vi "Read Calculation Results.vi"(0 "VISA resource name":refnum<visa-resource-name>, 5 "Calculate Option (0: Read Math Calculation)":i32(ring) items=["Read Math Calculation", "Recalculate Math Calculation", "Read Buffer Data Calculation", "Read Limit Tests"], 11 "error in (no error)":errorcluster) -> (3 "Limit1 Test Failed":bool, 4 "VISA resource name out":refnum<visa-resource-name>, 6 "Math Calculation Result":string="0", 8 "Buffer Data Calculation Result":dbl format="%.6e", 10 "Composite Result":bool, 14 "Limit2 Test Failed":bool, 15 "error out":errorcluster)   [LabVIEW 2016, in "Keithley 6517.lvlib"]
doc: "Performs CALC 1, CALC2 or CALC3 calculate operation and reads the result.\n\n<B>Note:</B>\n(1) Composite Limit Result is not compatible with <B>model 6514</B>. When reading limit tests, Composite Limit Result will always reaad -1 indicating invalid or no data.\n(2) You must first enable selected calculation (CALC1, CALC2, or CALC3) and run <B>Initiate</B> VI in Low-level Data."
uses:
  <instrlib>/Keithley 6517/Keithley 6517.lvlib
panel:
  # "Limit Tests Results"
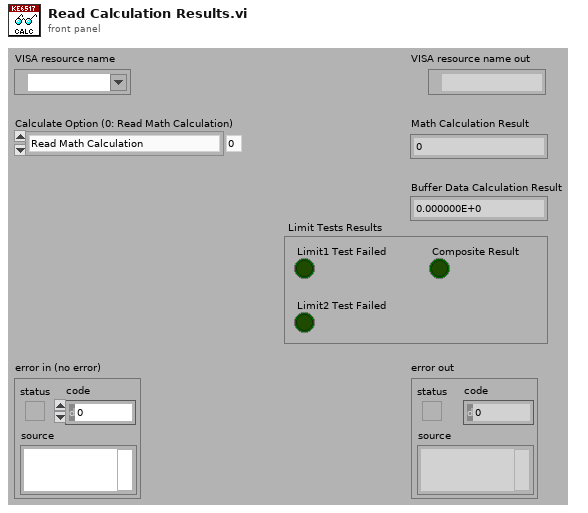
[diagram p1: front panel]
types:
  T1 = typedef "Keithley 6517.lvlib/Extended User Data.ctl" = cluster{"Instrument Model":i32}
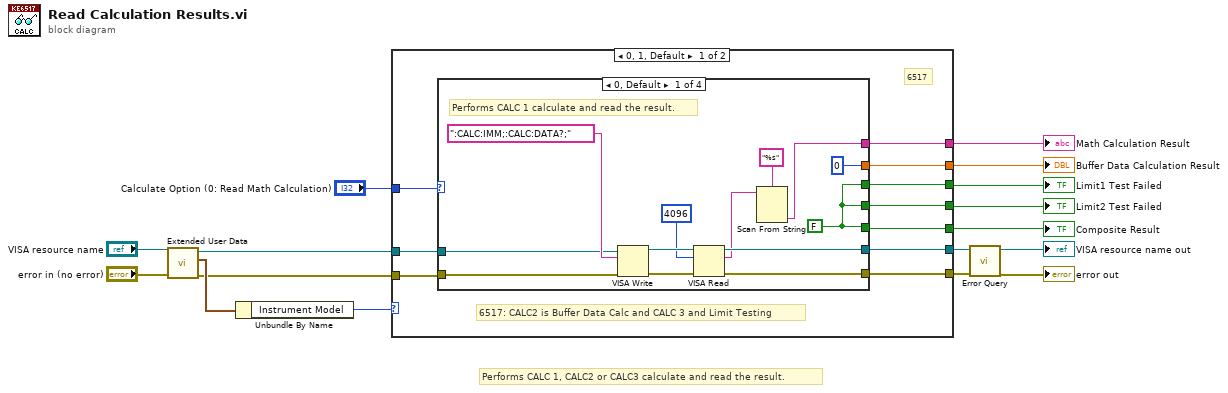
[diagram p0: block diagram]
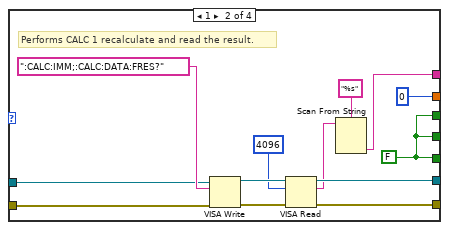
[diagram p2: hidden frame]
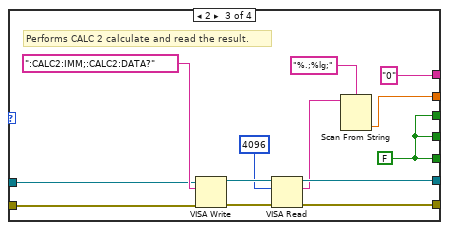
[diagram p3: hidden frame]
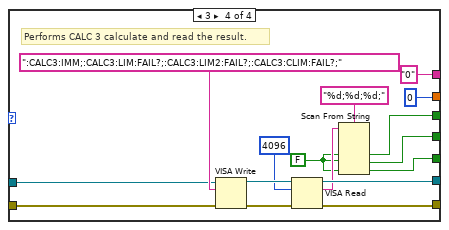
[diagram p4: hidden frame]
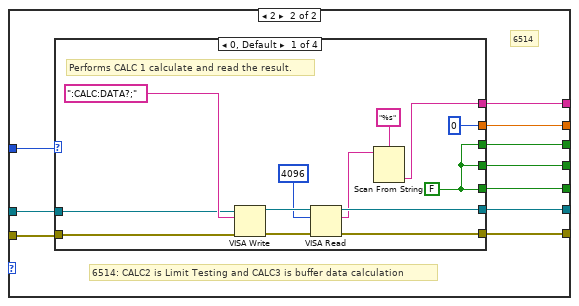
[diagram p5: hidden frame]
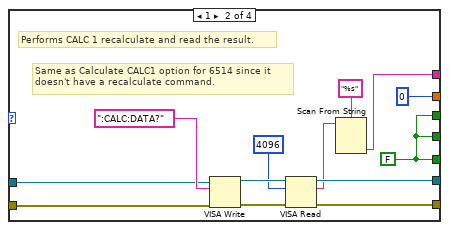
[diagram p6: hidden frame]
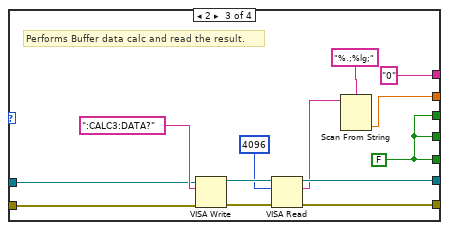
[diagram p7: hidden frame]
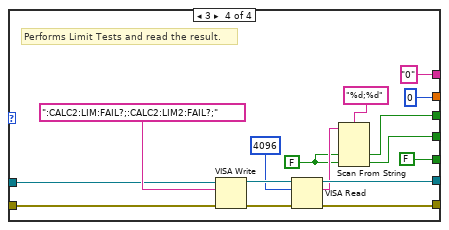
[diagram p8: hidden frame]
diagram:
  # "Performs CALC 1, CALC2 or CALC3 calculate and read the result."
  n1 = call <instrlib>:"Extended User Data.vi"("error in (no error)"="error in (no error)", "VISA resource name"="VISA resource name") -> ("error out"=w9:errorcluster, "User Data Out"=w10:T1, "VISA resource name out"=w8:refnum<visa-resource-name>)  [unwired: 7 in]
  n2 = Unbundle By Name(w10) -> ("Instrument Model"=w7:i32)
  n3 = case shown="0, 1, Default" w7 {
    tunnel: "Calculate Option (0: Read Math Calculation)" -> [w26 w91]
    tunnel: [w25 w90] -> w13
    tunnel: [w24 w89] -> w12
    tunnel: [w23 w88] -> w11
    tunnel: [w22 w87] -> w4
    tunnel: w9 -> [w21 w86]
    tunnel: w8 -> [w20 w85]
    tunnel: [w19 w84] -> w3
    tunnel: [w18 w83] -> w2
    tunnel: [w17 w82] -> w1
    frame 0, 1, Default {
      # "6517"
      # "6517: CALC2 is Buffer Data Calc and CALC 3 and Limit Testing"
      n4 = case shown="0, Default" w26 {
        tunnel: w21 -> [w34 w47 w60 w76]
        tunnel: [w33 w46 w59 w75] -> w25
        tunnel: [w32 w45 w58 w74] -> w24
        tunnel: [w31 w44 "0" "0"] -> w23
        tunnel: [0 0 w55 0] -> w22
        tunnel: w20 -> [w28 w41 w54 w70]
        tunnel: [w27 w40 w53 w68] -> w19
        tunnel: [w27 w40 w53 w67] -> w18
        tunnel: [w27 w40 w53 w66] -> w17
        frame 0, Default {
          w27 = FALSE
          # "Performs CALC 1 calculate and read the result."
          n5 = VISA Write(VISA resource name=w28, write buffer=":CALC:IMM;:CALC:DATA?;", error in (no error)=w34) -> (VISA resource name out=w38:refnum<visa-resource-name>, error out=w39:errorcluster)  [unwired: 1 out]
          n6 = VISA Read(VISA resource name=w38, byte count=u32 4096, error in (no error)=w39) -> (VISA resource name out=w33:refnum<visa-resource-name>, read buffer=w29:string, error out=w32:errorcluster)  [unwired: 1 out]
          n7 = Scan From String(format string="%s", input string=w29) -> (output 1=w31:string)  [unwired: 3 in, 3 out]
        }
        frame 1 {
          w40 = FALSE
          # "Performs CALC 1 recalculate and read the result."
          n8 = VISA Write(VISA resource name=w41, write buffer=":CALC:IMM;:CALC:DATA:FRES?", error in (no error)=w47) -> (VISA resource name out=w51:refnum<visa-resource-name>, error out=w52:errorcluster)  [unwired: 1 out]
          n9 = VISA Read(VISA resource name=w51, byte count=u32 4096, error in (no error)=w52) -> (VISA resource name out=w46:refnum<visa-resource-name>, read buffer=w42:string, error out=w45:errorcluster)  [unwired: 1 out]
          n10 = Scan From String(format string="%s", input string=w42) -> (output 1=w44:string)  [unwired: 3 in, 3 out]
        }
        frame 2 {
          w53 = FALSE
          # "Performs CALC 2 calculate and read the result."
          n11 = VISA Write(VISA resource name=w54, write buffer=":CALC2:IMM;:CALC2:DATA?", error in (no error)=w60) -> (VISA resource name out=w64:refnum<visa-resource-name>, error out=w65:errorcluster)  [unwired: 1 out]
          n12 = VISA Read(VISA resource name=w64, byte count=u32 4096, error in (no error)=w65) -> (VISA resource name out=w59:refnum<visa-resource-name>, read buffer=w57:string, error out=w58:errorcluster)  [unwired: 1 out]
          n13 = Scan From String(format string="%.;%lg;", input string=w57) -> (output 1=w55:dbl)  [unwired: 3 in, 3 out]
        }
        frame 3 {
          w69 = FALSE
          # "Performs CALC 3 calculate and read the result."
          n14 = VISA Write(VISA resource name=w70, write buffer=":CALC3:IMM;:CALC3:LIM:FAIL?;:CALC3:LIM2:FAIL?;:CALC3:CLIM:FAIL?;", error in (no error)=w76) -> (VISA resource name out=w80:refnum<visa-resource-name>, error out=w81:errorcluster)  [unwired: 1 out]
          n15 = VISA Read(VISA resource name=w80, byte count=u32 4096, error in (no error)=w81) -> (VISA resource name out=w75:refnum<visa-resource-name>, read buffer=w71:string, error out=w74:errorcluster)  [unwired: 1 out]
          n16 = Scan From String(format string="%d;%d;%d;", input string=w71, default 1=w69, default 2=w69, default 3=w69) -> (output 1=w68:bool, output 2=w67:bool, output 3=w66:bool)  [unwired: 2 in, 3 out]
        }
      }
    }
    frame 2 {
      # "6514"
      # "6514: CALC2 is Limit Testing and CALC3 is buffer data calculation"
      n17 = case shown="0, Default" w91 {
        tunnel: w86 -> [w94 w106 w125 w141]
        tunnel: [w99 w112 w124 w140] -> w90
        tunnel: [w98 w111 w123 w139] -> w89
        tunnel: [w97 w110 "0" "0"] -> w88
        tunnel: [0 0 w120 0] -> w87
        tunnel: w85 -> [w93 w107 w119 w135]
        tunnel: [w92 w105 w118 w133] -> w84
        tunnel: [w92 w105 w118 w132] -> w83
        tunnel: [w92 w105 w118 FALSE] -> w82
        frame 0, Default {
          w92 = FALSE
          # "Performs CALC 1 calculate and read the result."
          n18 = VISA Write(VISA resource name=w93, write buffer=":CALC:DATA?;", error in (no error)=w94) -> (VISA resource name out=w103:refnum<visa-resource-name>, error out=w104:errorcluster)  [unwired: 1 out]
          n19 = VISA Read(VISA resource name=w103, byte count=u32 4096, error in (no error)=w104) -> (VISA resource name out=w99:refnum<visa-resource-name>, read buffer=w95:string, error out=w98:errorcluster)  [unwired: 1 out]
          n20 = Scan From String(format string="%s", input string=w95) -> (output 1=w97:string)  [unwired: 3 in, 3 out]
        }
        frame 1 {
          w105 = FALSE
          # "Same as Calculate CALC1 option for 6514 since it\ndoesn't have a recalculate command."
          # "Performs CALC 1 recalculate and read the result."
          n21 = VISA Write(VISA resource name=w107, write buffer=":CALC:DATA?", error in (no error)=w106) -> (VISA resource name out=w116:refnum<visa-resource-name>, error out=w117:errorcluster)  [unwired: 1 out]
          n22 = VISA Read(VISA resource name=w116, byte count=u32 4096, error in (no error)=w117) -> (VISA resource name out=w112:refnum<visa-resource-name>, read buffer=w108:string, error out=w111:errorcluster)  [unwired: 1 out]
          n23 = Scan From String(format string="%s", input string=w108) -> (output 1=w110:string)  [unwired: 3 in, 3 out]
        }
        frame 2 {
          w118 = FALSE
          # "Performs Buffer data calc and read the result."
          n24 = VISA Write(VISA resource name=w119, write buffer=":CALC3:DATA?", error in (no error)=w125) -> (VISA resource name out=w129:refnum<visa-resource-name>, error out=w130:errorcluster)  [unwired: 1 out]
          n25 = VISA Read(VISA resource name=w129, byte count=u32 4096, error in (no error)=w130) -> (VISA resource name out=w124:refnum<visa-resource-name>, read buffer=w122:string, error out=w123:errorcluster)  [unwired: 1 out]
          n26 = Scan From String(format string="%.;%lg;", input string=w122) -> (output 1=w120:dbl)  [unwired: 3 in, 3 out]
        }
        frame 3 {
          w134 = FALSE ("default value 2")
          # "Performs Limit Tests and read the result."
          n27 = VISA Write(VISA resource name=w135, write buffer=":CALC2:LIM:FAIL?;:CALC2:LIM2:FAIL?;", error in (no error)=w141) -> (VISA resource name out=w145:refnum<visa-resource-name>, error out=w146:errorcluster)  [unwired: 1 out]
          n28 = VISA Read(VISA resource name=w145, byte count=u32 4096, error in (no error)=w146) -> (VISA resource name out=w140:refnum<visa-resource-name>, read buffer=w136:string, error out=w139:errorcluster)  [unwired: 1 out]
          n29 = Scan From String(format string="%d;%d", input string=w136, default 1=w134, default 2=w134) -> (output 1=w133:bool, output 2=w132:bool)  [unwired: 2 in, 3 out]
        }
      }
    }
  }
  "Buffer Data Calculation Result" <- w4
  "Math Calculation Result" <- w11
  "Limit1 Test Failed" <- w3
  "Limit2 Test Failed" <- w2
  "Composite Result" <- w1
  n30 = call <instrlib>:"Error Query.vi"("error in (no error)"=w12, "VISA resource name"=w13) -> ("error out"=→"error out":errorcluster, "VISA resource name out"=→"VISA resource name out":refnum<visa-resource-name>)  [unwired: 6 in, 2 out]
